vi "getZkAndDofInGroups.vi"(8 "error in (no error)":errorcluster, 11 "OptStateEsti in":refnum<class "OptStateEsti.lvclass">) -> (0 "error out":errorcluster, 1 "DOF in Groups":T1, 2 "zn3Idx":bool[](array[boolean]), 3 "OptStateEsti out":refnum<class "OptStateEsti.lvclass">)   [LabVIEW 2016, in "OfcFunc.lvlib" / "OptStateEsti.lvclass"]
doc: "Get the index array of Zk and DOF in groups (M2 hexapod, camera hexapod, M1M3 bending mode, M2 bending mode)."
uses:
  OptStateEsti.lvclass
  StrictDef/DofGroup.ctl
  OptStateEsti.lvclass/OptStateEsti.ctl
  OfcFunc.lvlib
  MatOper/MatOper.lvclass
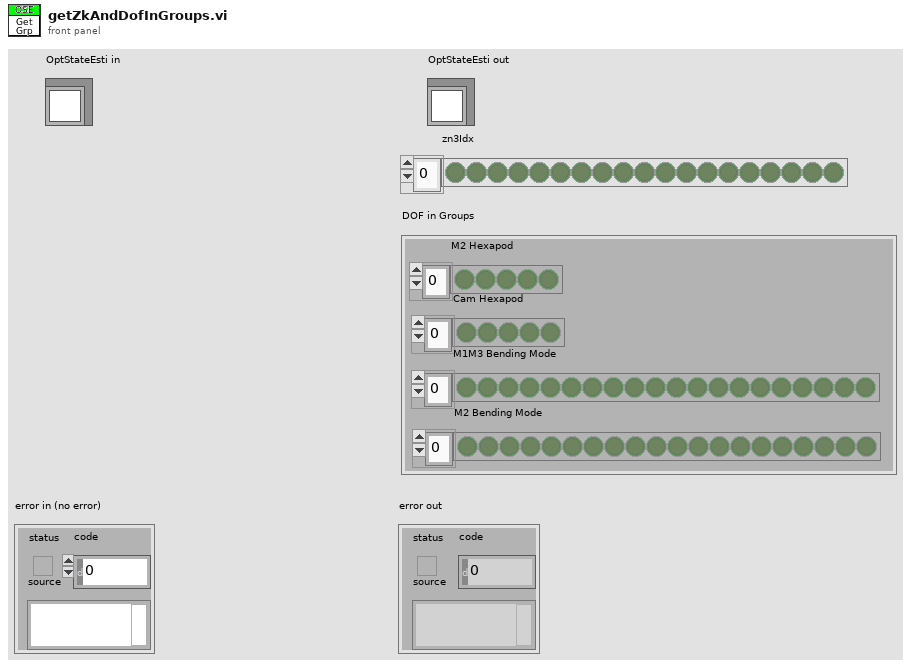
[diagram p1: front panel]
types:
  T1 = cluster{"M2 Hexapod":bool[], "Cam Hexapod ":bool[], "M1M3 Bending Mode":bool[], "M2 Bending Mode":bool[]}
  T2 = typedef "OfcFunc.lvlib/DofGroup.ctl" = enum16{"M2 Hex Pos", "Cam Hex Pos", "M1M3 Bend", "M2 Bend"}
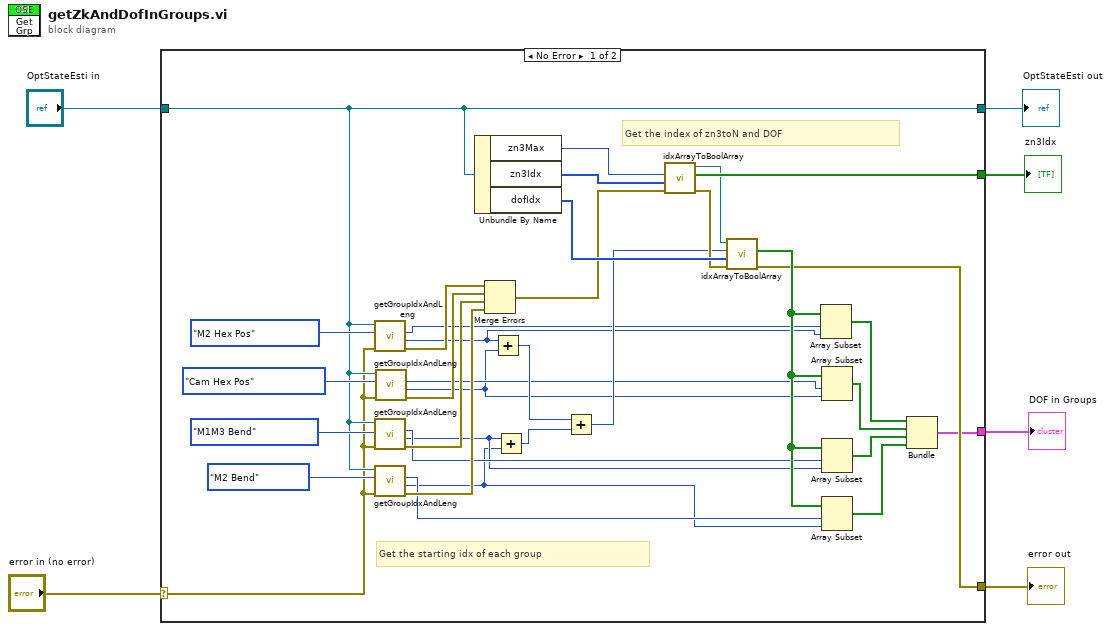
[diagram p0: block diagram]
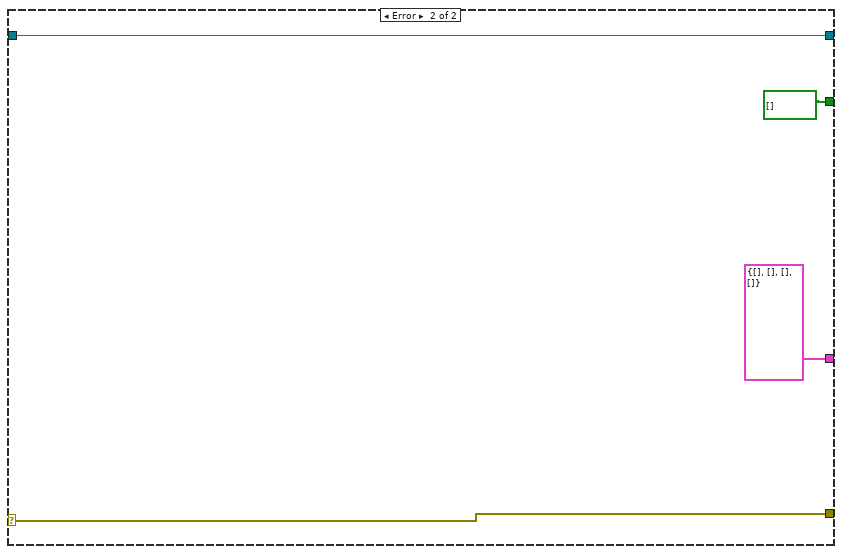
[diagram p2: hidden frame]
diagram:
  n1 = case shown="No Error" "error in (no error)" {
    selector: "error in (no error)" -> [w21 w45]
    tunnel: [w36 w45] -> w6
    tunnel: [w25 w44] -> w5
    tunnel: "OptStateEsti in" -> [w25 w44]
    tunnel: [w31 cluster{bool[], bool[], bool[], bool[]} {[], [], [], []}] -> w3
    tunnel: [w30 bool[] [] ("Bool Array")] -> w2
    frame No Error {
      # "Get the index of zn3toN and DOF"
      # "Get the starting idx of each group"
      n2 = call "getGroupIdxAndLeng.vi"("error in (no error)"=w21, "DOF Group"=DofGroup."M2 Hex Pos", "OptStateEsti in"=w25) -> ("error out"=w17:errorcluster, "Group Length"=w11:i32, "Start Index"=w15:i32)  [unwired: 5 in, 1 out]
      n3 = call "getGroupIdxAndLeng.vi"("error in (no error)"=w21, "DOF Group"=DofGroup."M1M3 Bend", "OptStateEsti in"=w25) -> ("error out"=w19:errorcluster, "Group Length"=w9:i32, "Start Index"=w13:i32)  [unwired: 5 in, 1 out]
      n4 = call "getGroupIdxAndLeng.vi"("error in (no error)"=w21, "DOF Group"=DofGroup."M2 Bend", "OptStateEsti in"=w25) -> ("error out"=w20:errorcluster, "Group Length"=w8:i32, "Start Index"=w12:i32)  [unwired: 5 in, 1 out]
      n5 = call "getGroupIdxAndLeng.vi"("error in (no error)"=w21, "DOF Group"=DofGroup."Cam Hex Pos", "OptStateEsti in"=w25) -> ("error out"=w18:errorcluster, "Group Length"=w10:i32, "Start Index"=w14:i32)  [unwired: 5 in, 1 out]
      n6 = Unbundle By Name(w25) -> ("zn3Max"=w37:i32, "zn3Idx"=w38:i32[], "dofIdx"=w40:i32[])
      n7 = Merge Errors(w17, w18, w19, w20) -> (w16:errorcluster)
      n8 = Add(x=w11, y=w10) -> (x+y=w23:i32)
      n9 = Add(x=w9, y=w8) -> (x+y=w24:i32)
      n10 = Add(x=w23, y=w24) -> (x+y=w22:i32)
      n11 = call "idxArrayToBoolArray.vi"("error in (no error)"=w16, "Idx Array"=w38, "Length of Bool Array"=w37) -> ("error out"=w39:errorcluster, "Bool Array"=w30:bool[], "MatOper out"=w7:refnum<class "MatOper.lvclass">)  [unwired: 6 in]
      n12 = call "idxArrayToBoolArray.vi"("error in (no error)"=w39, "Idx Array"=w40, "Length of Bool Array"=w22, "MatOper in"=w7) -> ("error out"=w36:errorcluster, "Bool Array"=w41:bool[])  [unwired: 5 in, 1 out]
      n13 = Array Subset(array=w41, index=w15, length=w11) -> (w35:bool[])
      n14 = Array Subset(array=w41, index=w14, length=w10) -> (w34:bool[])
      n15 = Array Subset(array=w41, index=w13, length=w9) -> (w33:bool[])
      n16 = Array Subset(array=w41, index=w12, length=w8) -> (w32:bool[])
      n17 = Bundle(w35, w34, w33, w32) -> (w31:cluster{bool[], bool[], bool[], bool[]})  [unwired: 1 in]
    }
    frame Error {
    }
  }
  "error out" <- w6
  "OptStateEsti out" <- w5
  "DOF in Groups" <- w3
  "zn3Idx" <- w2
